vi "Wave2D_Init Data.vi"(0 "F(t, x, y)":dbl[][][](array[numeric]), 1 "Initial Value":dbl[][](array[numeric]), 2 "Initial Derivative":dbl[][](array[numeric]), 5 "k":dbl=1.0, 7 "a":dbl, 9 "Domain":T2={"t"={"initial t"=0.0, "final t"=1.0, "# of t-points"=11}, "x"={"start x"=0.0, "end x"=1.0, "# of x-points"=11}, "y"={"start y"=0.0, "end y"=1.0, "# of y-points"=11}}, 12 "Boundary Condition":cluster{"type":T1, "Value":dbl[][]}[](array[cluster]) {"type" items=["Dirichlet", "Neumann"]}) -> (4 "Wave2D Data":T3={"PDE"={"k"=0.0, "a"=0.0, "F(t, x, y)"=[]}, "Domain"={"t"={"initial t"=0.0, "final t"=0.0, "# of t-points"=0}, "x"={"start x"=0.0, "end x"=0.0, "# of x-points"=0}, "y"={"start y"=0.0, "end y"=1.0, "# of y-points"=11}, "delta"={"delta t"=0.0, "delta x"=0.0, "delta y"=0.0}}, "BC"={"Start X"={"type"=0, "Value"=[]}, "End X"={"type"=0, "Value"=[]}, "Start Y"={"type"=0, "Value"=[]}, "End Y"={"type"=0, "Value"=[]}}, "Corner"={"Start X & Start Y"=[], "Start X & End Y"=[], "End X & Start Y"=[], "End X & End Y"=[]}, "IC"={"Value"=[], "Derivative"=[]}, "P"={"Sub Diag"=[], "Diag"=[], "Super Diag"=[], "P"=[]}, "LU of P"={"L"=[], "U"={"Diag"=[], "Super Diag"=[], "2nd Super Diag"=[]}, "Pivot"=[]}, "Q"={"Sub Diag"=[], "Diag"=[], "Super Diag"=[], "Q"=[]}, "LU of Q"={"L"=[], "U"={"Diag"=[], "Super Diag"=[], "2nd Super Diag"=[]}, "Pivot"=[]}, "State"={"U"=[], "Old U"=[], "V&W"=[], "x start index"=0, "x length"=0, "y start index"=0, "y length"=0}} {"BC"."End Y"."type" items=["Dirichlet", "Neumann"]; "BC"."Start Y"."type" items=["Dirichlet", "Neumann"]; "BC"."End X"."type" items=["Dirichlet", "Neumann"]; "BC"."Start X"."type" items=["Dirichlet", "Neumann"]})   [LabVIEW 2017, in "NI_PDE.lvlib"]
uses:
  <vilib>/gmath/NI_PDE.lvlib
  <vilib>/gmath/pde.llb/Wave2D/Wave2D_Data.ctl
  <vilib>/gmath/pde.llb/Common/PDE_BC Type.ctl
  <vilib>/Analysis/Matrix/Datatypes/RealMatrix.ctl
  <vilib>/Analysis/Matrix/NI_Matrix.lvlib
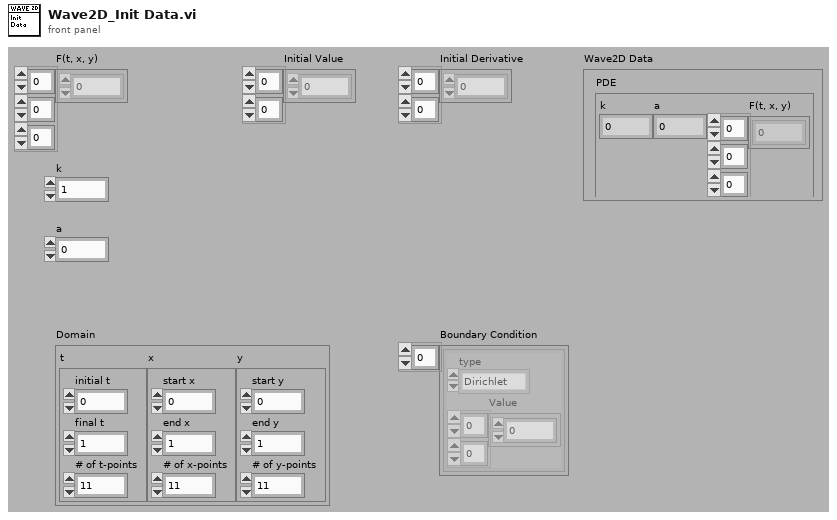
[diagram p1: front panel]
types:
  T1 = typedef "NI_PDE.lvlib/PDE_BC Type.ctl" = i32
  T2 = cluster{"t":cluster{"initial t":dbl, "final t":dbl, "# of t-points":i32}, "x":cluster{"start x":dbl, "end x":dbl, "# of x-points":i32}, "y":cluster{"start y":dbl, "end y":dbl, "# of y-points":i32}}
  T3 = typedef "NI_PDE.lvlib/Wave2D_Data.ctl" = cluster{"PDE":cluster{"k":dbl, "a":dbl, "F(t, x, y)":dbl[][][]}, "Domain":cluster{"t":cluster{"initial t":dbl, "final t":dbl, "# of t-points":i32}, "x":cluster{"start x":dbl, "end x":dbl, "# of x-points":i32}, "y":cluster{"start y":dbl, "end y":dbl, "# of y-points":i32}, "delta":cluster{"delta t":dbl, "delta x":dbl, "delta y":dbl}}, "BC":cluster{"Start X":cluster{"type":T1, "Value":dbl[][]}, "End X":cluster{"type":T1, "Value":dbl[][]}, "Start Y":cluster{"type":T1, "Value":dbl[][]}, "End Y":cluster{"type":T1, "Value":dbl[][]}}, "Corner":cluster{"Start X & Start Y":dbl[], "Start X & End Y":dbl[], "End X & Start Y":dbl[], "End X & End Y":dbl[]}, "IC":cluster{"Value":dbl[][], "Derivative":dbl[][]}, "P":cluster{"Sub Diag":dbl[], "Diag":dbl[], "Super Diag":dbl[], "P":T4}, "LU of P":cluster{"L":dbl[], "U":cluster{"Diag":dbl[], "Super Diag":dbl[], "2nd Super Diag":dbl[]}, "Pivot":i32[]}, "Q":cluster{"Sub Diag":dbl[], "Diag":dbl[], "Super Diag":dbl[], "Q":T4}, "LU of Q":cluster{"L":dbl[], "U":cluster{"Diag":dbl[], "Super Diag":dbl[], "2nd Super Diag":dbl[]}, "Pivot":i32[]}, "State":cluster{"U":dbl[][], "Old U":dbl[][], "V&W":dbl[][], "x start index":i32, "x length":i32, "y start index":i32, "y length":i32}}
  T4 = typedef "NI_Matrix.lvlib/RealMatrix.ctl" = dbl[][]
  T5 = cluster{"Start X & Start Y":dbl[], "Start X & End Y":dbl[], "End X & Start Y":dbl[], "End X & End Y":dbl[]}
  T6 = cluster{"Start X":cluster{"type":T1, "Value":dbl[][]}, "End X":cluster{"type":T1, "Value":dbl[][]}, "Start Y":cluster{"type":T1, "Value":dbl[][]}, "End Y":cluster{"type":T1, "Value":dbl[][]}}
  T7 = cluster{"L":dbl[], "U":cluster{"Diag":dbl[], "Super Diag":dbl[], "2nd Super Diag":dbl[]}, "Pivot":i32[]}
  T8 = cluster{"Sub Diag":dbl[], "Diag":dbl[], "Super Diag":dbl[], "A":T4}
  T9 = cluster{"initial t":dbl, "final t":dbl, "# of t-points":i32}
  T10 = cluster{"start x":dbl, "end x":dbl, "# of x-points":i32}
  T11 = cluster{"start y":dbl, "end y":dbl, "# of y-points":i32}
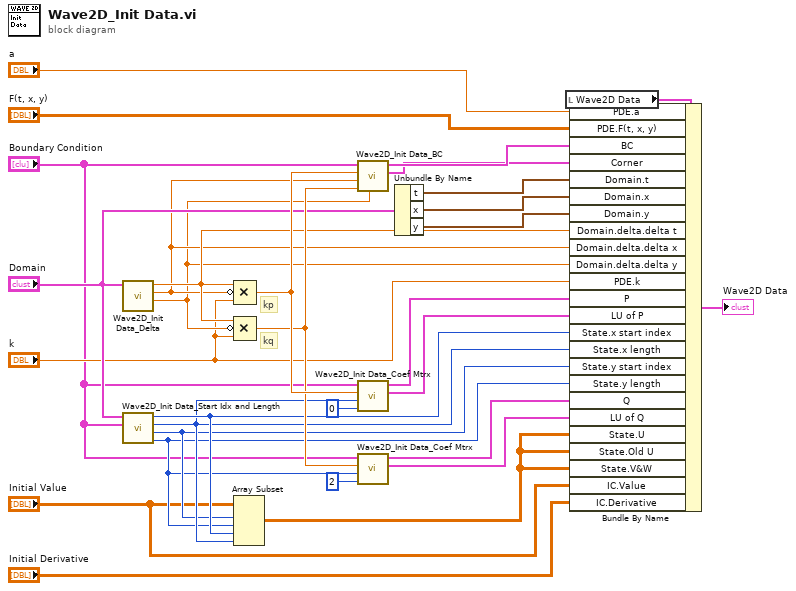
[diagram p0: block diagram]
diagram:
  # "kq"
  # "kp"
  n1 = call <vilib>:"Wave2D_Init Data_Delta.vi"("Domain"="Domain") -> ("delta y"=w16:dbl, "delta x"=w17:dbl, "delta t"=w18:dbl)  [unwired: 8 out]
  n2 = call <vilib>:"Wave2D_Init Data_Start Idx and Length.vi"("Boundary Condition"="Boundary Condition", "Domain"="Domain") -> ("y length"=w5:i32, "y start index"=w6:i32, "x length"=w7:i32, "x start index"=w8:i32)  [unwired: 6 out]
  n3 = Compound Arithmetic op=MULTIPLY(w18, invert w17, "k") -> (w30:dbl)
  n4 = Compound Arithmetic op=MULTIPLY(w18, invert w16, "k") -> (w27:dbl)
  n5 = Array Subset(array="Initial Value", index (row)=w6, length (row)=w5, index (col)=w8, length (col)=w7) -> (w9:dbl[][])
  n6 = call <vilib>:"Wave2D_Init Data_BC.vi"("delta y"=w16, "kq"=w27, "delta x"=w17, "kp"=w30, "Boundary Condition"="Boundary Condition") -> ("Corner"=w23:T5, "BC"=w25:T6)  [unwired: 5 out]
  n7 = call <vilib>:"Wave2D_Init Data_Coef Mtrx.vi"("BC start index"=0, "length"=w7, "ks"=w30, "Boundary Condition"="Boundary Condition") -> ("LU of A"=w15:T7, "A"=w12:T8)  [unwired: 6 out]
  n8 = call <vilib>:"Wave2D_Init Data_Coef Mtrx.vi"("BC start index"=2, "length"=w5, "ks"=w27, "Boundary Condition"="Boundary Condition") -> ("LU of A"=w13:T7, "A"=w14:T8)  [unwired: 6 out]
  n9 = Unbundle By Name("Domain") -> ("t"=w21:T9, "x"=w20:T10, "y"=w19:T11)
  n10 = local read "Wave2D Data"() -> (w29:T3)
  n11 = Bundle By Name(cluster=w29, "PDE.a"="a", "PDE.F(t, x, y)"="F(t, x, y)", "BC"=w25, "Corner"=w23, "Domain.t"=w21, "Domain.x"=w20, "Domain.y"=w19, "Domain.delta.delta t"=w18, "Domain.delta.delta x"=w17, "Domain.delta.delta y"=w16, "PDE.k"="k", "P"=w12, "LU of P"=w15, "State.x start index"=w8, "State.x length"=w7, "State.y start index"=w6, "State.y length"=w5, "Q"=w14, "LU of Q"=w13, "State.U"=w9, "State.Old U"=w9, "State.V&W"=w9, "IC.Value"="Initial Value", "IC.Derivative"="Initial Derivative") -> (→"Wave2D Data":T3)
